vi "parse ID byte.vi"(10 "ID byte":string) -> (0 "Output?":bool, 1 "Input?":bool, 2 "Node ID":u32, 3 "Enum":enum16{""}(ring))   [LabVIEW 2011]
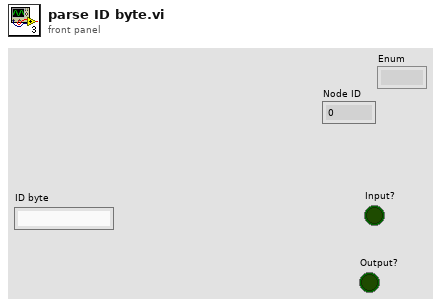
[diagram p1: front panel]
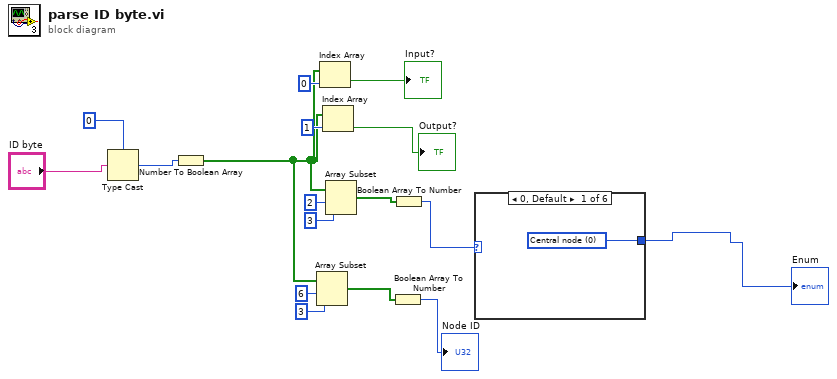
[diagram p0: block diagram]
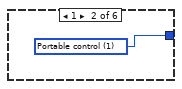
[diagram p2: hidden frame]
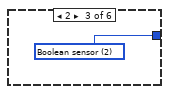
[diagram p3: hidden frame]
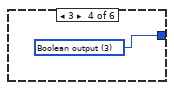
[diagram p4: hidden frame]
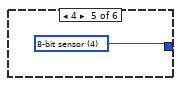
[diagram p5: hidden frame]
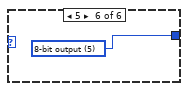
[diagram p6: hidden frame]
diagram:
  n1 = Type Cast(type=0, x="ID byte") -> (*(type *) &x=w15:i32)
  n2 = Number To Boolean Array(number=w15) -> (Boolean array=w10:bool[])
  n3 = Array Subset(array=w10, index=6, length=3) -> (w3:bool[])
  n4 = Index Array(array=w10, index=0) -> (element=→"Input?":bool)
  n5 = Index Array(array=w10, index=1) -> (element=→"Output?":bool)
  n6 = Array Subset(array=w10, index=2, length=3) -> (w5:bool[])
  n7 = Boolean Array To Number(Boolean array=w3) -> (number=→"Node ID":u32)
  n8 = Boolean Array To Number(Boolean array=w5) -> (number=w4:u32)
  n9 = case shown="0, Default" w4 {
    tunnel: [w18 w19 w20 w21 w22 w23] -> w1
    frame 0, Default {
      w18 = u16 0 items=["Central node", "Portable control", "Boolean sensor", "Boolean output", "8-bit sensor", "8-bit output"] ("Type")
    }
    frame 1 {
      w19 = u16 1 items=["Central node", "Portable control", "Boolean sensor", "Boolean output", "8-bit sensor", "8-bit output"] ("Type")
    }
    frame 2 {
      w20 = u16 2 items=["Central node", "Portable control", "Boolean sensor", "Boolean output", "8-bit sensor", "8-bit output"] ("Type")
    }
    frame 3 {
      w21 = u16 3 items=["Central node", "Portable control", "Boolean sensor", "Boolean output", "8-bit sensor", "8-bit output"] ("Type")
    }
    frame 4 {
      w22 = u16 4 items=["Central node", "Portable control", "Boolean sensor", "Boolean output", "8-bit sensor", "8-bit output"] ("Type")
    }
    frame 5 {
      w23 = u16 5 items=["Central node", "Portable control", "Boolean sensor", "Boolean output", "8-bit sensor", "8-bit output"] ("Type")
    }
  }
  "Enum" <- w1
